vi "SugarCane_VM.vi"() -> ()   [LabVIEW 2017]
uses:
  Cluster_Settings.ctl
panel:
  in  "Enter The amount":dbl
  in  "PUSH":bool
  # "SUGARCANE JUICE\n                   RS 30"
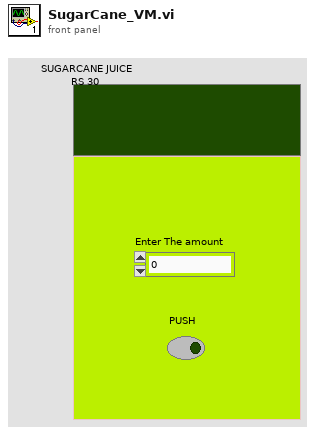
[diagram p1: front panel]
types:
  T1 = typedef "Cluster_Settings.ctl" = cluster{"No of cans":dbl, "Entered amount\n":dbl}
  T2 = enum16{"Initialize", "Waiting", "Check above 50", "Dispense", "Check for change", "Exit"}
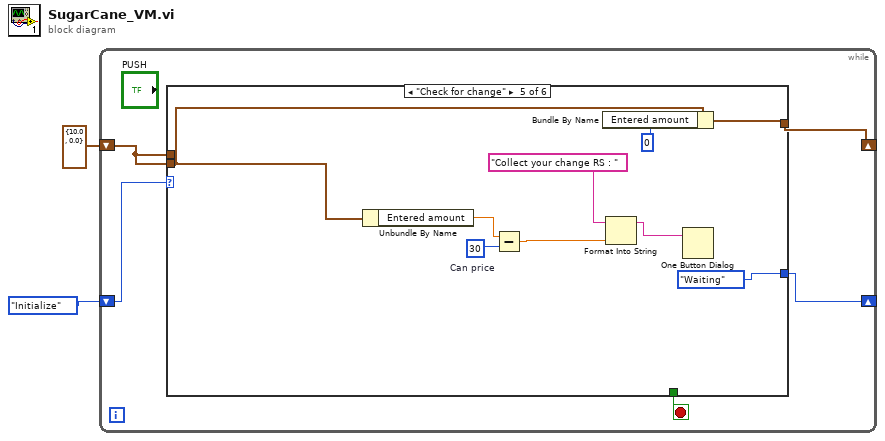
[diagram p0: block diagram]
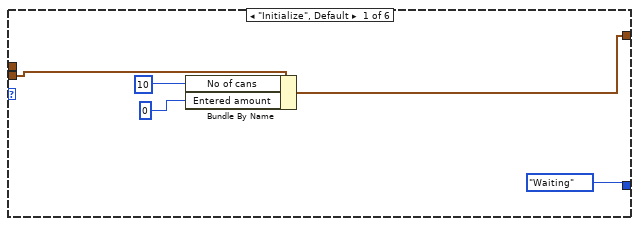
[diagram p2: hidden frame]
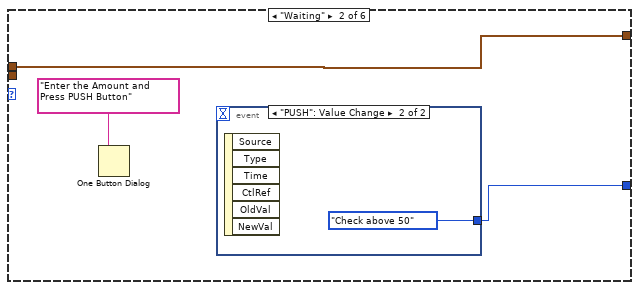
[diagram p3: hidden frame]
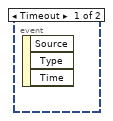
[diagram p4: hidden frame]
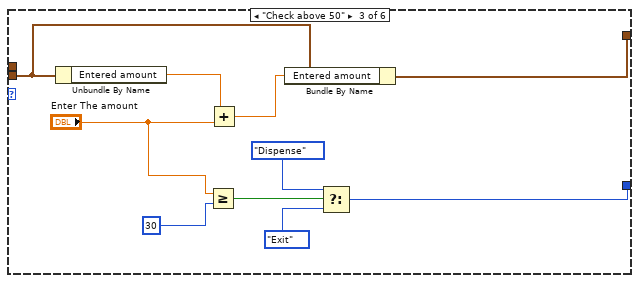
[diagram p5: hidden frame]
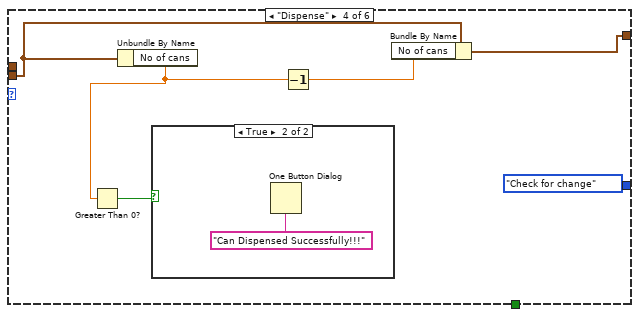
[diagram p6: hidden frame]
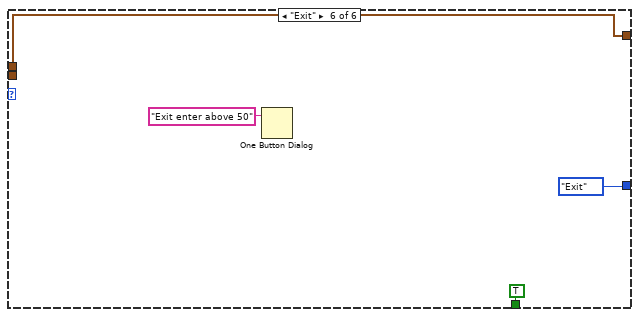
[diagram p8: hidden frame]
diagram:
  n1 = while {
    shift-right: [w5] -> _
    shift-left: T1 {"No of cans"=10.0, "Entered amount\n"=0.0} ("Cluster") -> [w4]
    shift-right: [w7] -> _
    shift-left: T2."Initialize" ("Enum-TypeDef") -> [w3]
    stop <- w6 stop-if-true
    n2 = case shown="\"Check for change\"" w3 {
      tunnel: w4 -> [w8 _ w22 w30 w39 w44]
      tunnel: [_ _ _ _ _ TRUE] -> w6
      tunnel: [T2."Waiting" ("Enum-TypeDef") w14 w19 T2."Check for change" ("Enum-TypeDef") T2."Waiting" ("Enum-TypeDef") T2."Exit" ("Enum-TypeDef")] -> w7
      tunnel: [w10 w13 w21 w29 w38 w44] -> w5
      tunnel: w4 -> [_ w13 _ _ _ _]
      frame "Initialize", Default {
        n3 = Bundle By Name "Bundle By Name"(cluster=w8, "No of cans"=10, "Entered amount"=0) -> (w10:T1)
      }
      frame "Waiting" {
        n4 = One Button Dialog(message="Enter the Amount and Press PUSH Button") -> ()  [unwired: 1 in, 1 out]
        n5 = event shown="[1] \"PUSH\": Value Change" {
          selector: _ -> [_ _]
          dyn-events: _ -> [_ _]
          timeout: _ -> [_ _]
          tunnel: [_ T2."Check above 50" ("Enum-TypeDef")] -> w14
          event Timeout {
            n6 = event-data() -> ()  [unwired: 1 in, 3 out]
          }
          event "PUSH": Value Change {
            n7 = event-data() -> ()  [unwired: 1 in, 6 out]
          }
        }
      }
      frame "Check above 50" {
        n8 = Unbundle By Name "Unbundle By Name"(w22) -> ("Entered amount"=w26:dbl)
        n9 = Greater Or Equal?(x="Enter The amount", y=30) -> (x >= y?=w23:bool)
        n10 = Add(x=w26, y="Enter The amount") -> (x+y=w20:dbl)
        n11 = Bundle By Name "Bundle By Name"(cluster=w22, "Entered amount"=w20) -> (w21:T1)
        n12 = Select(t=T2."Dispense" ("Enum-TypeDef"), s=w23, f=T2."Exit" ("Enum-TypeDef")) -> (s? t:f=w19:T2)
      }
      frame "Dispense" {
        n13 = Unbundle By Name "Unbundle By Name"(w30) -> ("No of cans"=w32:dbl)
        n14 = Greater Than 0?(x=w32) -> (x > 0?=w31:bool)
        n15 = case shown="True" w31 {
          frame False {
          }
          frame True {
            n16 = One Button Dialog(message="Can Dispensed Successfully!!!") -> ()  [unwired: 1 in, 1 out]
          }
        }
        n17 = Decrement(x=w32) -> (x-1=w28:dbl)
        n18 = Bundle By Name "Bundle By Name"(cluster=w30, "No of cans"=w28) -> (w29:T1)
      }
      frame "Check for change" {
        w41 = 30  # Can price
        n19 = Unbundle By Name "Unbundle By Name"(w39) -> ("Entered amount"=w42:dbl)
        n20 = Subtract(x=w42, y=w41) -> (x-y=w40:dbl)
        n21 = Bundle By Name "Bundle By Name"(cluster=w39, "Entered amount"=0) -> (w38:T1)
        n22 = Format Into String "Format Into String"(initial string="Collect your change RS : ", w40) -> (resulting string=w35:string)  [unwired: 2 in, 1 out]
        n23 = One Button Dialog(message=w35) -> ()  [unwired: 1 in, 1 out]
      }
      frame "Exit" {
        n24 = One Button Dialog(message="Exit enter above 50") -> ()  [unwired: 1 in, 1 out]
      }
    }
  }
